vi "Calculate_Cost_F()-3.vi"(0 "[IN] Subtracks":T2(array[cluster]), 1 "[IN] Still connected\ntracks in group":T1, 2 "[IN] Max angle":dbl, 3 "[IN] Areas particles\nPrimary Detected":dbl[][](array[numeric]), 7 "[IN] Index of Earliest \nProblem Point Inside":i32, 9 "[IN] # of Longest track\nInside the Tracks Group":i32, 11 "error IN":errorcluster, 12 "[IN] Primary \n(X,Y) Detected":dbl[][](array[numeric]), 13 "[IN] Potentially\nMoving (X,Y)":dbl[][](array[numeric]), 14 "[IN] Dot matrix with statuses \nfor potentially moving dots":i16[][](array[numeric])) -> (4 "[OUT] Cost function":i8[](array[numeric]), 15 "error OUT":errorcluster)   [LabVIEW 2013]
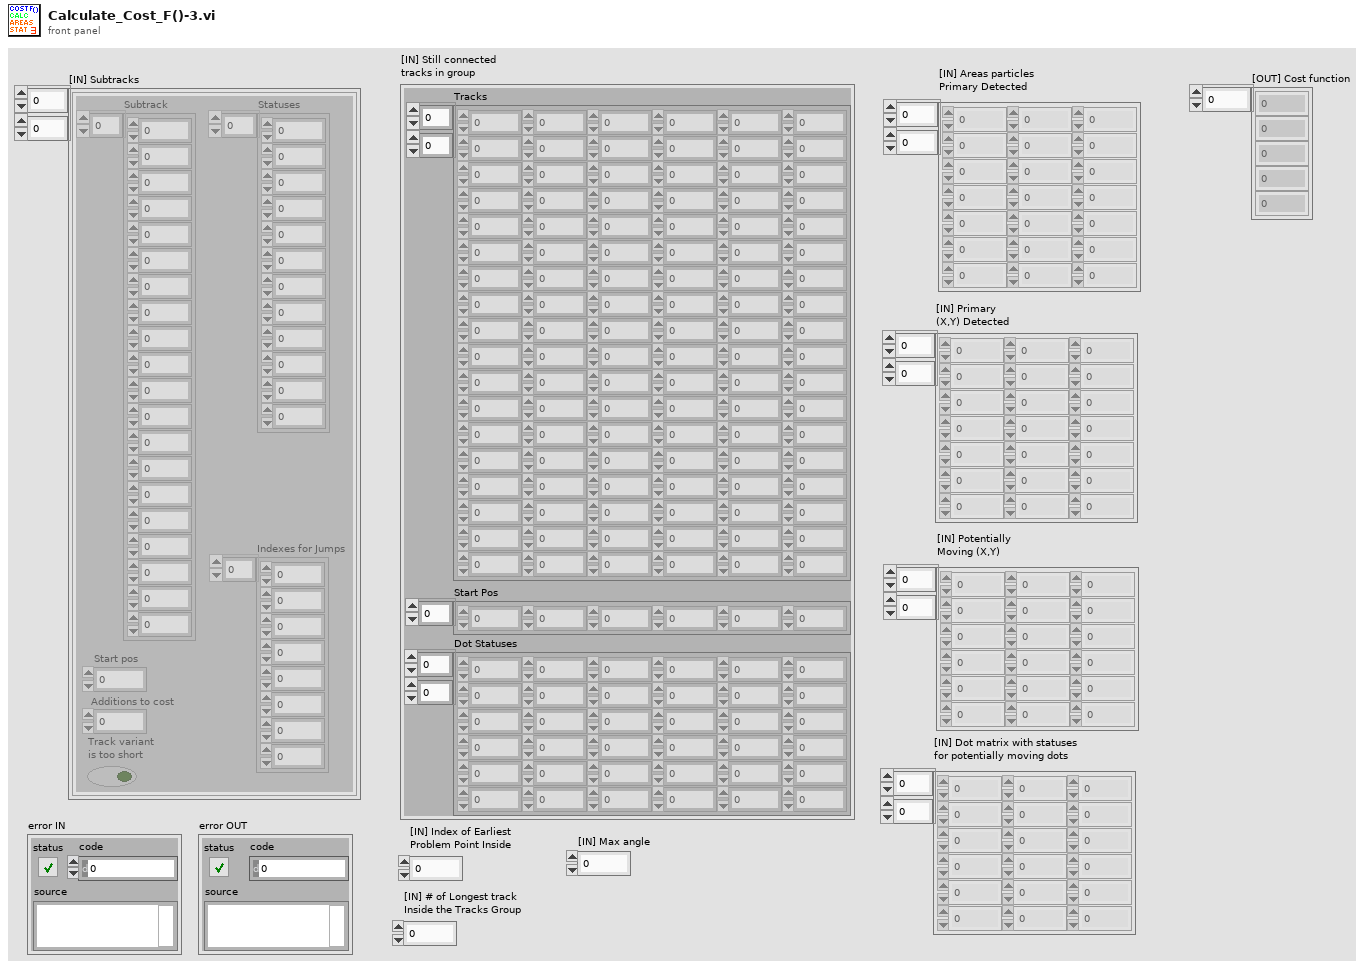
[diagram p1: front panel]
types:
  T1 = cluster{"Tracks":dbl[][], "Start Pos":i32[], "Dot Statuses":i16[][]}
  T2 = cluster{"Subtrack":dbl[], "Statuses":i16[], "Start pos":i32, "Additions to cost":i32, "Track variant \nis too short":bool, "Indexes for Jumps":i32[]}[][]
  T3 = cluster{"Subtrack":dbl[], "Statuses":i16[], "Start pos":i32, "Additions to cost":i32, "Track variant \nis too short":bool, "Indexes for Jumps":i32[]}[]
  T4 = cluster{"Subtrack":dbl[], "Statuses":i16[], "Start pos":i32, "Additions to cost":i32, "Track variant \nis too short":bool, "Indexes for Jumps":i32[]}
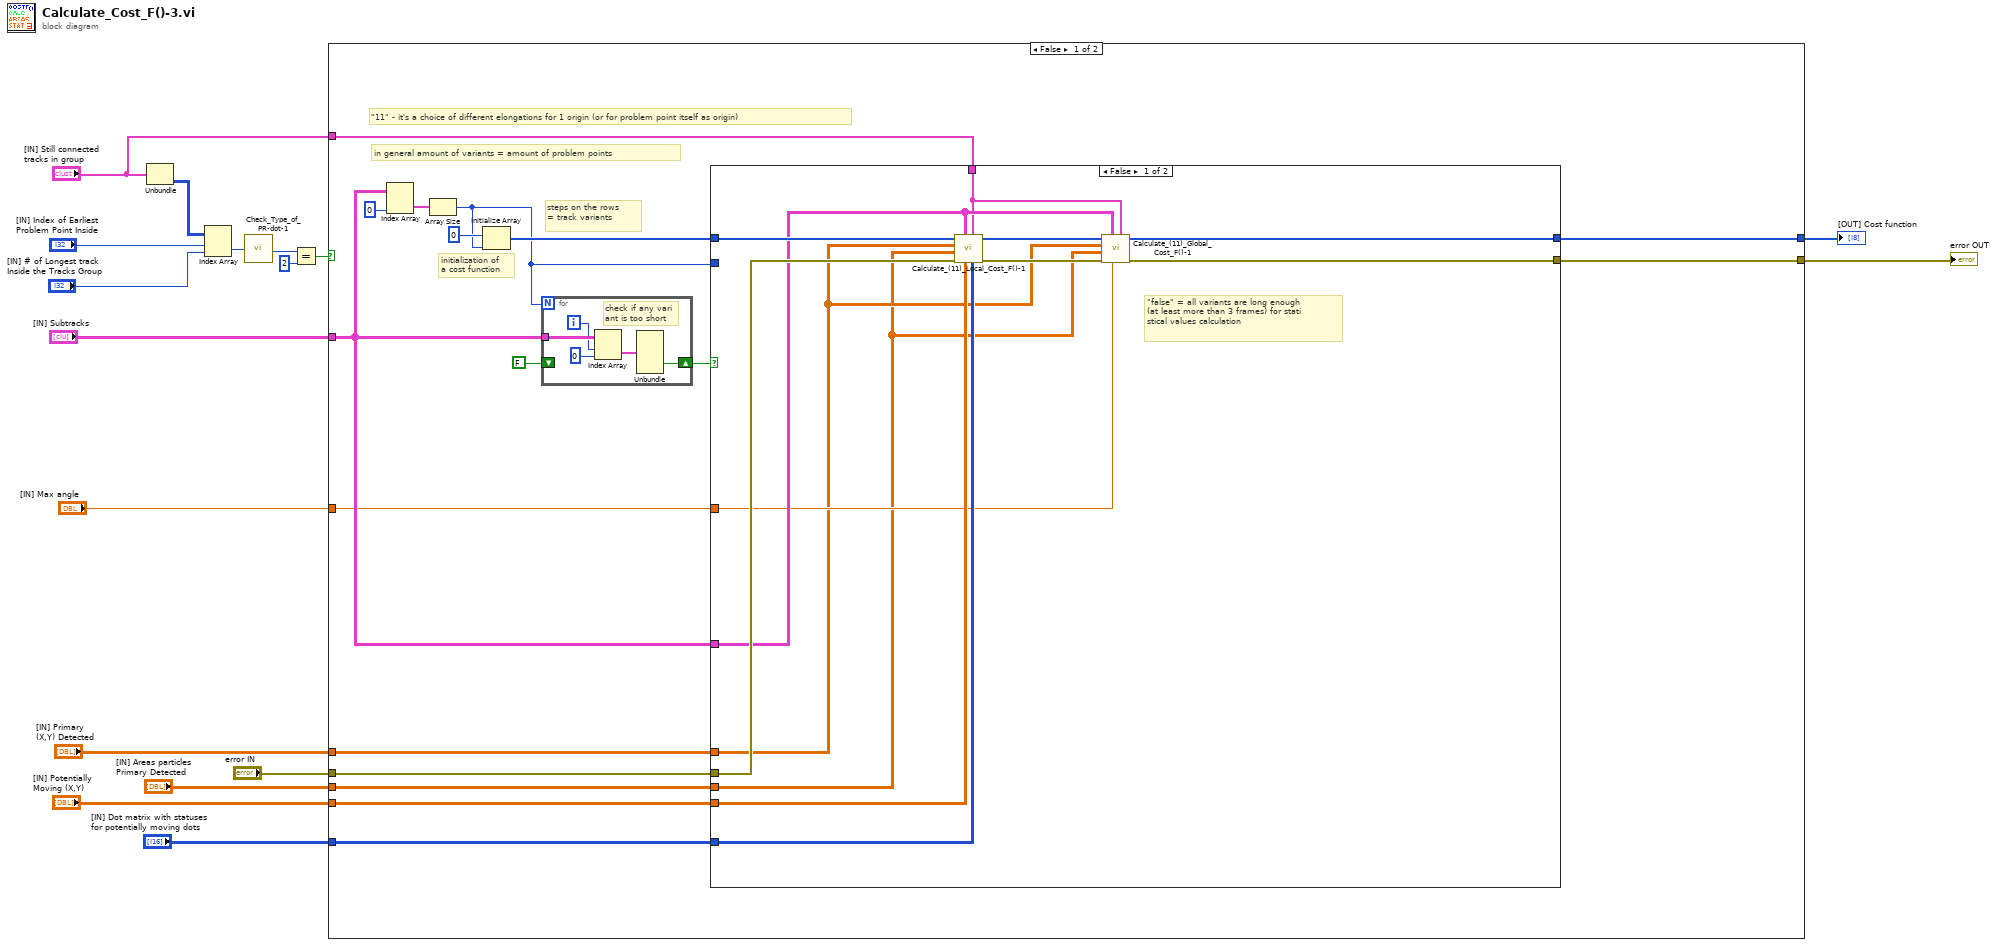
[diagram p0: block diagram]
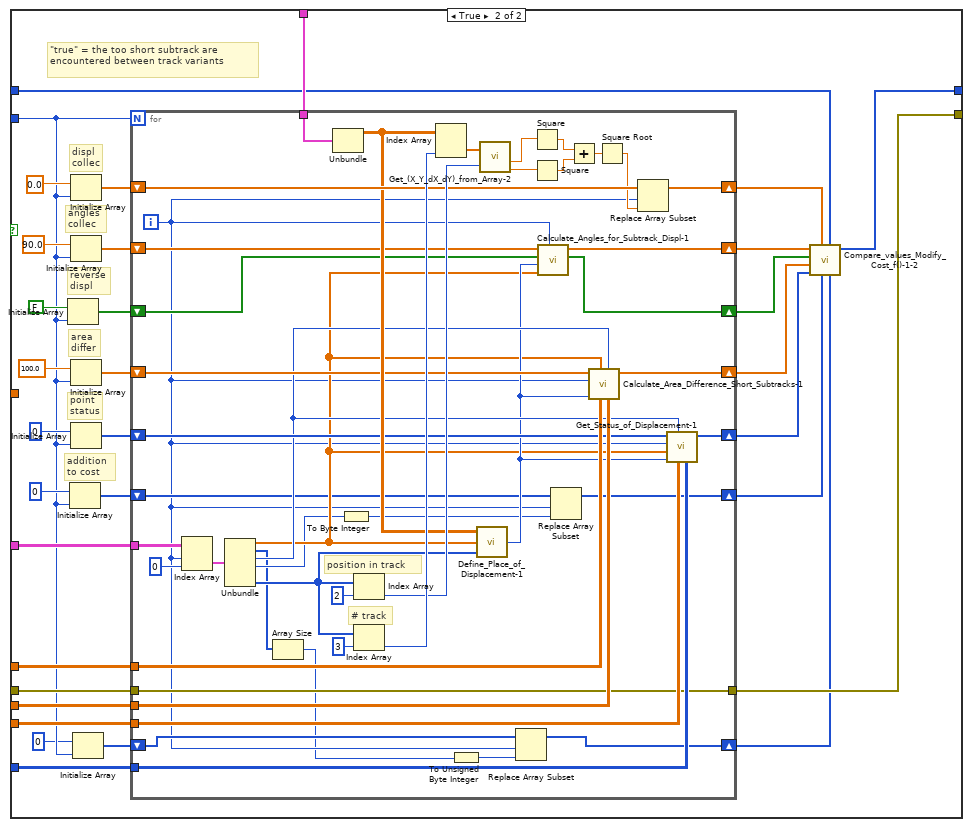
[diagram p2: hidden frame]
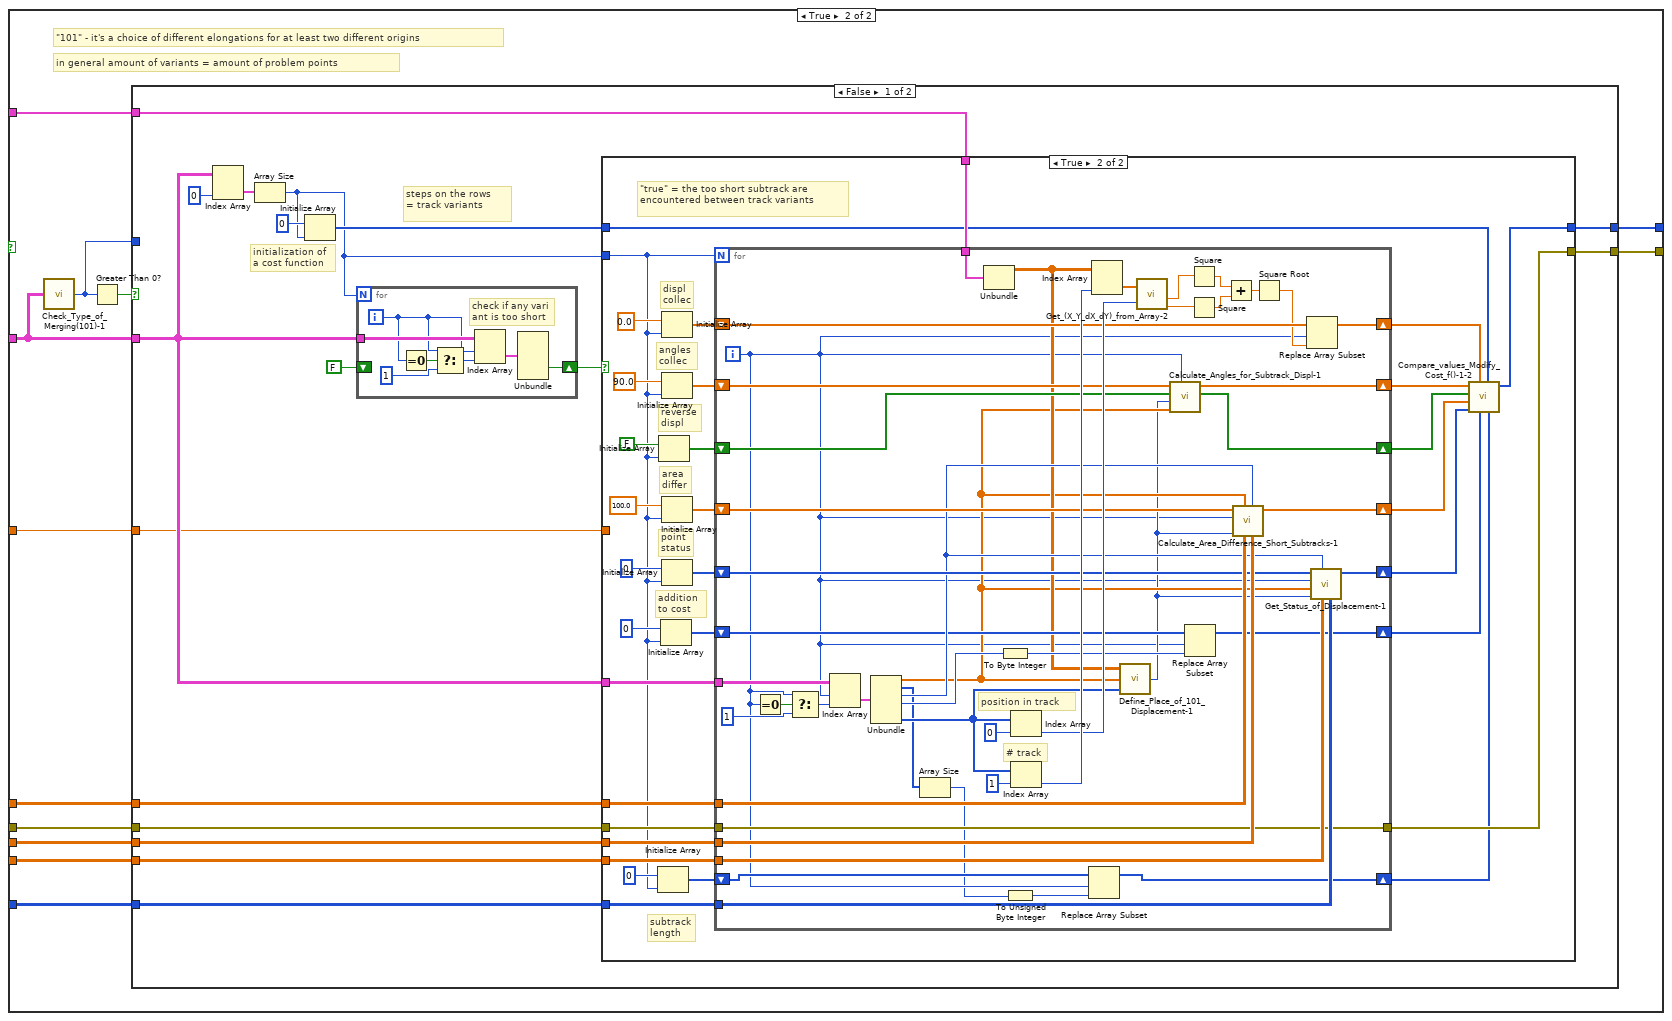
[diagram p3: hidden frame]
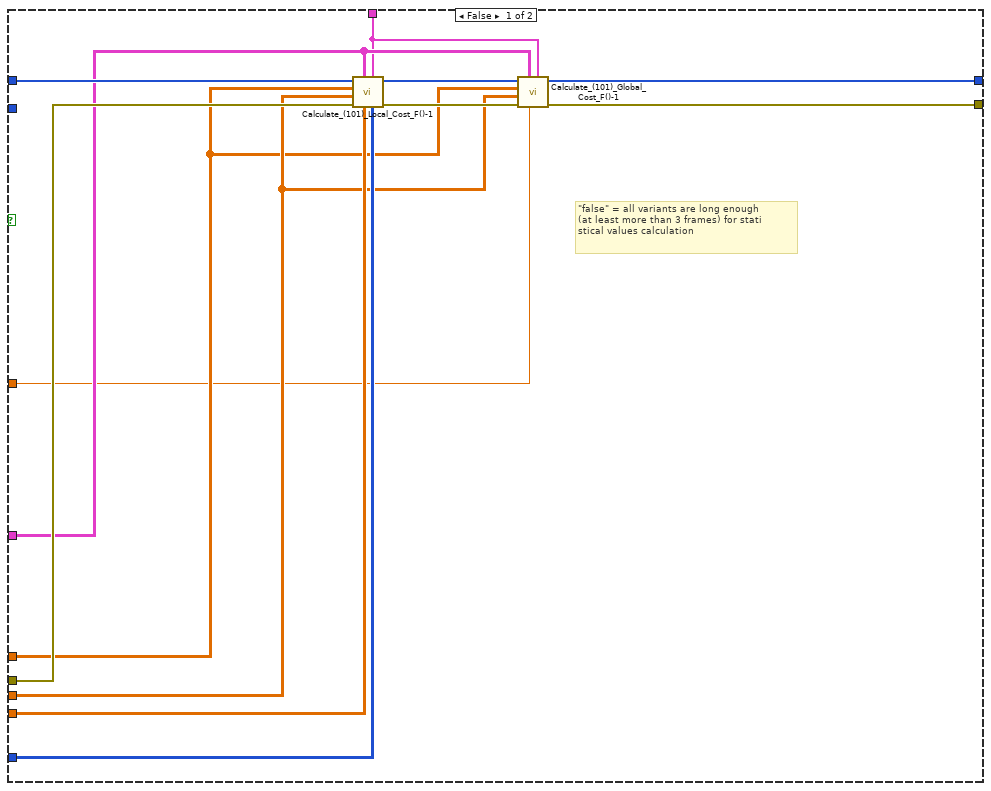
[diagram p4: hidden frame]
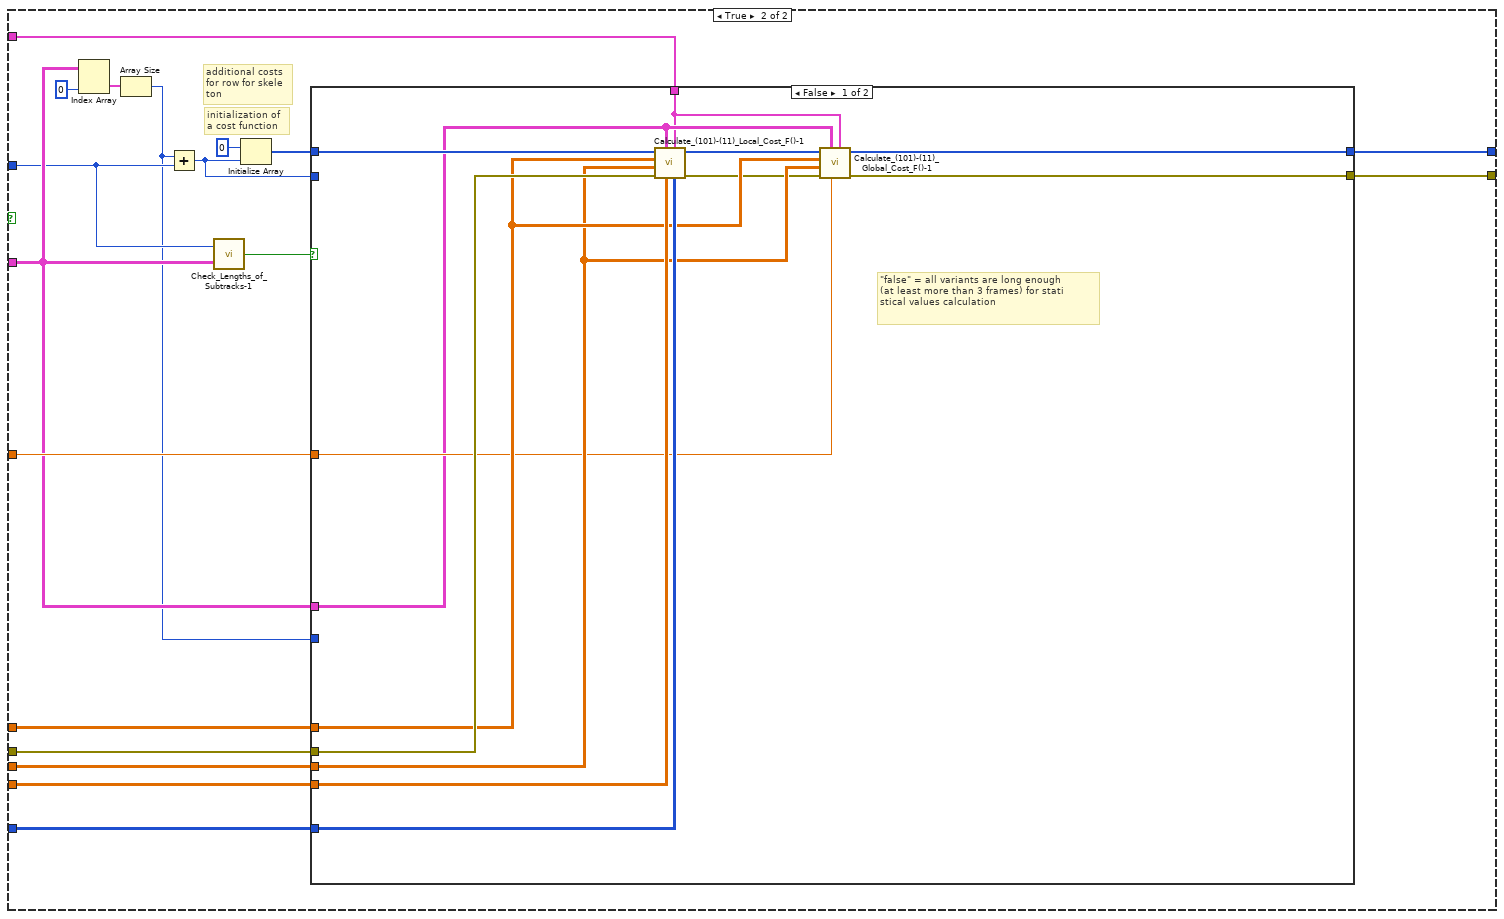
[diagram p5: hidden frame]
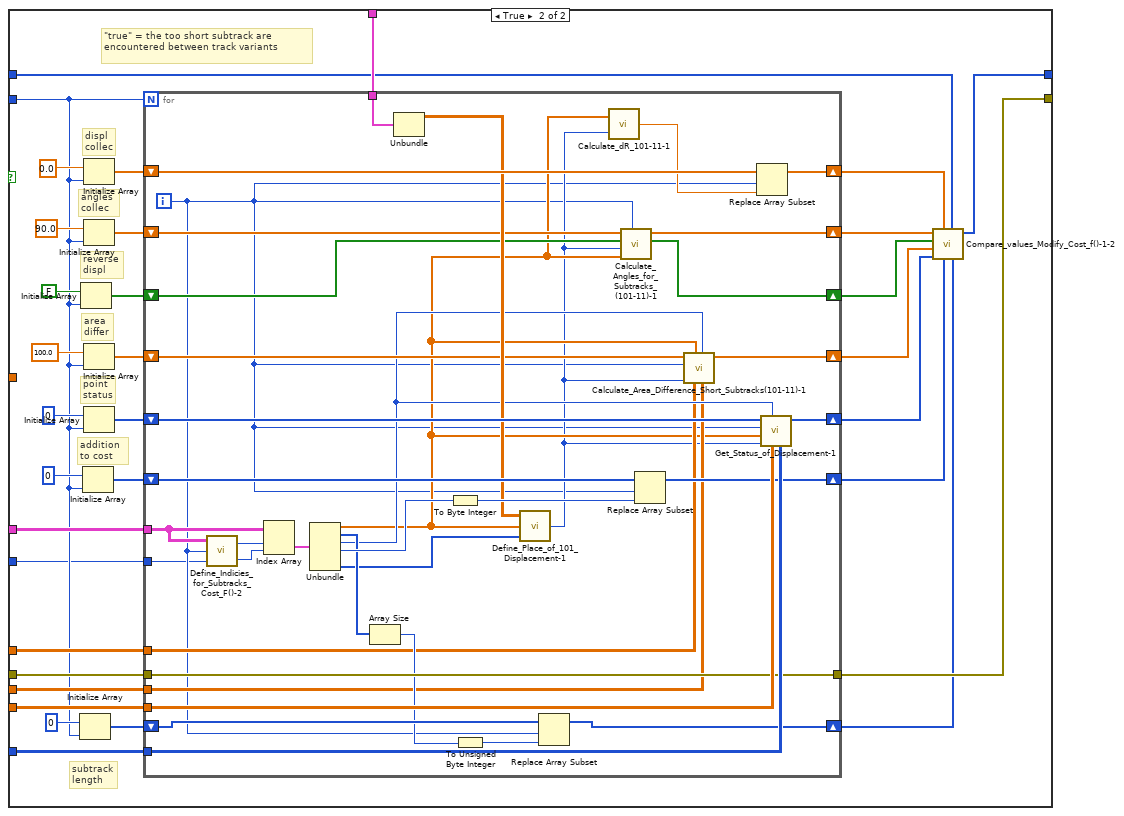
[diagram p6: hidden frame]
diagram:
  n1 = Unbundle("[IN] Still connected\ntracks in group") -> ("Dot Statuses"=w15:i16[][])  [unwired: 2 out]
  n2 = Index Array(array=w15, index (row)="[IN] Index of Earliest \nProblem Point Inside", index (col)="[IN] # of Longest track\nInside the Tracks Group") -> (element=w14:i16)
  n3 = call "Check_Type_of_PR-dot-1.vi"("[IN] dot status"=w14) -> ("[OUT] Type of\nproblem dot"=w17:i32)
  n4 = Equal?(x=w17, y=2) -> (x = y?=w13:bool)
  n5 = case shown="False" w13 {
    tunnel: "[IN] Subtracks" -> [w27 w133]
    tunnel: "[IN] Still connected\ntracks in group" -> [w26 w130]
    tunnel: "[IN] Primary \n(X,Y) Detected" -> [w25 w140]
    tunnel: "[IN] Areas particles\nPrimary Detected" -> [w24 w138]
    tunnel: "[IN] Potentially\nMoving (X,Y)" -> [w23 w137]
    tunnel: "[IN] Dot matrix with statuses \nfor potentially moving dots" -> [w22 w136]
    tunnel: "error IN" -> [w21 w139]
    tunnel: "[IN] Max angle" -> [w20 w141]
    tunnel: [w19 w135] -> w2
    tunnel: [w18 w134] -> w1
    frame False {
      # "initialization of \na cost function"
      # "steps on the rows\n= track variants"
      # "in general amount of variants = amount of problem points"
      # "\"11\" - it's a choice of different elongations for 1 origin (or for problem point itself as origin)"
      n6 = Index Array(array=w27, index (col)=0 ("disabled index (col)")) -> (element=w33:T3)  [unwired: 1 in]
      n7 = Array Size(array=w33) -> (size(s)=w28:i32)
      n8 = Initialize Array(i8 0, w28) -> (w29:i8[])
      n9 = for {
        N: w28 -> [_]
        tunnel: w27 -> [w129]
        shift-right: [w125] -> w30
        shift-left: FALSE -> [_]
        i -> [w126]
        # "check if any vari\nant is too short"
        n10 = Index Array(array=w129, index (row)=w126, index (col)=0 ("disabled index (col)")) -> (element=w127:T4)
        n11 = Unbundle(w127) -> ("Track variant \nis too short"=w125:bool)  [unwired: 5 out]
      }
      n12 = case shown="False" w30 {
        tunnel: w29 -> [w47 w54]
        tunnel: w28 -> [_ w59]
        tunnel: w27 -> [w42 w79]
        tunnel: w26 -> [w41 w78]
        tunnel: w25 -> [w38 w69]
        tunnel: w24 -> [w37 w68]
        tunnel: w23 -> [w45 w65]
        tunnel: w22 -> [w44 w64]
        tunnel: w21 -> [w46 w61]
        tunnel: w20 -> [w39 _]
        tunnel: [w36 w53] -> w19
        tunnel: [w35 w60] -> w18
        frame False {
          # "\"false\" = all variants are long enough\n(at least more than 3 frames) for stati\nstical values calculation"
          n13 = call "Calculate_(11)_Local_Cost_F()-1.vi"("[IN] Dot matrix with statuses \nfor potentially moving dots"=w44, "[IN] Still connected\ntracks in group"=w41, "[IN] Potentially\nMoving (X,Y)"=w45, "[IN] Subtracks"=w42, "error IN"=w46, "[IN] Areas particles\nPrimary Detected"=w37, "[IN] Primary \n(X,Y) Detected"=w38, "[IN] Cost function"=w47) -> ("error OUT"=w40:errorcluster, "[OUT] Cost function"=w43:i8[])  [unwired: 2 in]
          n14 = call "Calculate_(11)_Global_Cost_F()-1.vi"("[IN] Still connect\ned tracks in group"=w41, "[IN] Max angle"=w39, "[IN] Subtracks"=w42, "error IN"=w40, "[IN] Areas particles\nPrimary Detected"=w37, "[IN] Primary \n(X,Y) Detected"=w38, "[IN] Cost function"=w43) -> ("error OUT"=w35:errorcluster, "[OUT] Cost function"=w36:i8[])  [unwired: 3 in]
        }
        frame True {
          # "addition \nto cost"
          # "point\nstatus"
          # "area \ndiffer"
          # "reverse \ndispl"
          # "angles \ncollec"
          # "displ \ncollec"
          # "\"true\" = the too short subtrack are \nencountered between track variants"
          n15 = Initialize Array(FALSE, w59) -> (w72:bool[])
          n16 = Initialize Array(i8 0, w59) -> (w62:i8[])
          n17 = Initialize Array(0.0, w59) -> (w76:dbl[])
          n18 = Initialize Array(90.0, w59) -> (w74:dbl[])
          n19 = Initialize Array(100.0, w59) -> (w70:dbl[])
          n20 = Initialize Array(i16 0, w59) -> (w66:i16[])
          n21 = Initialize Array(u8 0, w59) -> (w57:u8[])
          n22 = for {
            N: w59 -> [_]
            tunnel: w79 -> [w124]
            tunnel: w78 -> [w119]
            shift-right: [w114] -> w55
            shift-left: w76 -> [w115]
            shift-right: [w110] -> w56
            shift-left: w74 -> [w111]
            shift-right: [w108] -> w52
            shift-left: w72 -> [w109]
            tunnel: w69 -> [w104]
            tunnel: w68 -> [w106]
            shift-right: [w105] -> w51
            shift-left: w70 -> [w107]
            tunnel: w65 -> [w99]
            tunnel: w64 -> [w98]
            shift-right: [w97] -> w50
            shift-left: w66 -> [w103]
            shift-right: [w93] -> w49
            shift-left: w62 -> [w96]
            tunnel: w61 -> [w86]
            tunnel: [w86] -> w60
            shift-right: [w83] -> w48
            shift-left: w57 -> [w84]
            i -> [w82]
            # "# track"
            # "position in track"
            n23 = Index Array(array=w124, index (row)=w82, index (col)=0 ("disabled index (col)")) -> (element=w122:T4)
            n24 = Unbundle(w122) -> ("Subtrack"=w100:dbl[], "Statuses"=w85:i16[], "Start pos"=w102:i32, "Additions to cost"=w95:i32, "Indexes for Jumps"=w112:i32[])  [unwired: 1 out]
            n25 = Array Size(array=w85) -> (size(s)=w81:i32)
            n26 = Unbundle(w119) -> ("Tracks"=w113:dbl[][])  [unwired: 2 out]
            n27 = To Byte Integer(number=w95) -> (8bit integer=w94:i8)
            n28 = Index Array(array=w112, index=2) -> (element=w116:i32)
            n29 = Index Array(array=w112, index=3) -> (element=w118:i32)
            n30 = Index Array(array=w113, index (col)=w118) -> (element=w117:dbl[])  [unwired: 1 in]
            n31 = To Unsigned Byte Integer(number=w81) -> (unsigned 8bit integer=w80:u8)
            n32 = call "Define_Place_of_Displacement-1.vi"("[IN] Indexes for Jumps"=w112, "[IN] Subtrack"=w100, "[IN] Tracks"=w113) -> ("[OUT] Index of \"11\" Dis\nplacement in Subtrack"=w101:i32)  [unwired: 2 in]
            n33 = call "Get_(X_Y_dX_dY)_from_Array-2.vi"("(X,Y,dX,dY)"=w117, "Index of Displacement"=w116) -> ("dX"=w89:dbl, "dY"=w88:dbl)  [unwired: 2 out]
            n34 = Replace Array Subset(array=w84, new element=w80, index=w82) -> (w83:u8[])
            n35 = Square(x=w89) -> (x^2=w92:dbl)
            n36 = Square(x=w88) -> (x^2=w91:dbl)
            n37 = call "Calculate_Angles_for_Subtrack_Displ-1.vi"("[IN] Index of subtrack"=w82, "[IN] Subtrack"=w100, "[IN] Index of \"11\" Dis-\nplacement in Subtrack"=w101, "[IN] Reverse Displ or Not"=w109, "[IN] Array with Angles \nBetween Displacement"=w111) -> ("[OUT] Reverse displacement or not"=w108:bool[], "[OUT] Angles betwe\nen two displacements"=w110:dbl[])  [unwired: 3 in]
            n38 = Replace Array Subset(array=w96, new element=w94, index=w82) -> (w93:i8[])
            n39 = Add(x=w92, y=w91) -> (x+y=w90:dbl)
            n40 = call "Calculate_Area_Difference_Short_Subtracks-1.vi"("[IN] Areas particles\nPrimary Detected"=w106, "[IN] Start pos"=w102, "[IN] Primary \n(X,Y) Detected"=w104, "[IN] Subtrack"=w100, "[IN] Index of \"11\" Dis-\nplacement in Subtrack"=w101, "[IN] Index of\n subtrack"=w82, "[IN] Areas \ndifference"=w107) -> ("[OUT] Areas \ndifference"=w105:dbl[])  [unwired: 4 in]
            n41 = Square Root(x=w90) -> (sqrt(x)=w87:dbl)
            n42 = Replace Array Subset(array=w115, new element=w87, index=w82) -> (w114:dbl[])
            n43 = call "Get_Status_of_Displacement-1.vi"("[IN] Dot matrix with statuses\nfor potentially moving dots"=w98, "[IN] Potentially\nMoving (X,Y)"=w99, "[IN] Start pos"=w102, "[IN] Index of Problem\nPoint in Subtrack"=w101, "[IN] Subtrack"=w100, "[IN] Index of\n subtrack"=w82, "[IN] Displace-\nment Statuses"=w103) -> ("[OUT] Displace\nment Statuses"=w97:i16[])  [unwired: 4 in]
          }
          n44 = call "Compare_values_Modify_Cost_f()-1-2.vi"("[IN] Track Length"=w48, "[IN] Cost function"=w54, "[IN] Additions to cost"=w49, "[IN] Array of displa\ncement differences"=w55, "[IN] Statuses of points"=w50, "[IN] Areas \ndifferences"=w51, "[IN] Reverse or not"=w52, "[IN] Angles betwe\nen displacements"=w56) -> ("[OUT] Cost function"=w53:i8[])  [unwired: 3 in]
        }
      }
    }
    frame True {
      # "in general amount of variants = amount of problem points"
      # "\"101\" - it's a choice of different elongations for at least two different origins"
      n45 = call "Check_Type_of_Merging(101)-1.vi"("[IN] Subtracks"=w133) -> ("[OUT] # of Additional Costs"=w131:i32)
      n46 = Greater Than 0?(x=w131) -> (x > 0?=w132:bool)
      n47 = case shown="False" w132 {
        tunnel: w130 -> [w151 w265]
        tunnel: w133 -> [w150 w264]
        tunnel: w141 -> [w149 w266]
        tunnel: w140 -> [w148 w271]
        tunnel: w139 -> [w147 w270]
        tunnel: w138 -> [w146 w269]
        tunnel: w137 -> [w145 w268]
        tunnel: w136 -> [w144 w267]
        tunnel: [w143 w259] -> w135
        tunnel: [w142 w258] -> w134
        tunnel: w131 -> [_ w261]
        frame False {
          # "initialization of \na cost function"
          # "steps on the rows\n= track variants"
          n48 = Index Array(array=w150, index (col)=0 ("disabled index (col)")) -> (element=w157:T3)  [unwired: 1 in]
          n49 = Array Size(array=w157) -> (size(s)=w152:i32)
          n50 = Initialize Array(i8 0, w152) -> (w153:i8[])
          n51 = for {
            N: w152 -> [_]
            tunnel: w150 -> [w257]
            shift-right: [w255] -> w154
            shift-left: FALSE -> [_]
            i -> [w251]
            # "check if any vari\nant is too short"
            n52 = Equal To 0?(x=w251) -> (x = 0?=w254:bool)
            n53 = Select(t=w251, s=w254, f=1) -> (s? t:f=w252:i32)
            n54 = Index Array(array=w257, index (row)=w251, index (col)=w252) -> (element=w256:T4)
            n55 = Unbundle(w256) -> ("Track variant \nis too short"=w255:bool)  [unwired: 5 out]
          }
          n56 = case shown="True" w154 {
            tunnel: w153 -> [w171 w178]
            tunnel: w152 -> [_ w182]
            tunnel: w150 -> [w163 w203]
            tunnel: w151 -> [w162 w202]
            tunnel: w148 -> [w165 w193]
            tunnel: w146 -> [w166 w192]
            tunnel: w145 -> [w170 w189]
            tunnel: w144 -> [w168 w188]
            tunnel: w147 -> [w169 w185]
            tunnel: w149 -> [w161 _]
            tunnel: [w160 w177] -> w143
            tunnel: [w159 w184] -> w142
            frame False {
              # "\"false\" = all variants are long enough\n(at least more than 3 frames) for stati\nstical values calculation"
              n57 = call "Calculate_(101)_Local_Cost_F()-1.vi"("[IN] Dot matrix with statuses \nfor potentially moving dots"=w168, "[IN] Still connected\ntracks in group"=w162, "[IN] Potentially\nMoving (X,Y)"=w170, "[IN] Subtracks"=w163, "error IN"=w169, "[IN] Areas particles\nPrimary Detected"=w166, "[IN] Primary \n(X,Y) Detected"=w165, "[IN] Cost function"=w171) -> ("error OUT"=w167:errorcluster, "[OUT] Cost function"=w164:i8[])  [unwired: 2 in]
              n58 = call "Calculate_(101)_Global_Cost_F()-1.vi"("[IN] Still connect\ned tracks in group"=w162, "[IN] Max angle"=w161, "[IN] Subtracks"=w163, "error IN"=w167, "[IN] Areas particles\nPrimary Detected"=w166, "[IN] Primary \n(X,Y) Detected"=w165, "[IN] Cost function"=w164) -> ("error OUT"=w159:errorcluster, "[OUT] Cost function"=w160:i8[])  [unwired: 3 in]
            }
            frame True {
              # "subtrack\nlength"
              # "addition \nto cost"
              # "point\nstatus"
              # "area \ndiffer"
              # "reverse \ndispl"
              # "angles \ncollec"
              # "displ \ncollec"
              # "\"true\" = the too short subtrack are \nencountered between track variants"
              n59 = Initialize Array(u8 0, w182) -> (w181:u8[])
              n60 = Initialize Array(FALSE, w182) -> (w196:bool[])
              n61 = Initialize Array(i8 0, w182) -> (w186:i8[])
              n62 = Initialize Array(0.0, w182) -> (w200:dbl[])
              n63 = Initialize Array(90.0, w182) -> (w198:dbl[])
              n64 = Initialize Array(100.0, w182) -> (w194:dbl[])
              n65 = Initialize Array(i16 0, w182) -> (w190:i16[])
              n66 = for {
                N: w182 -> [_]
                tunnel: w203 -> [w250]
                tunnel: w202 -> [w246]
                shift-right: [w241] -> w179
                shift-left: w200 -> [w242]
                shift-right: [w239] -> w180
                shift-left: w198 -> [w240]
                shift-right: [w237] -> w173
                shift-left: w196 -> [w238]
                tunnel: w193 -> [w233]
                tunnel: w192 -> [w235]
                shift-right: [w234] -> w174
                shift-left: w194 -> [w236]
                tunnel: w189 -> [w230]
                tunnel: w188 -> [w229]
                shift-right: [w228] -> w175
                shift-left: w190 -> [w232]
                shift-right: [w224] -> w176
                shift-left: w186 -> [w227]
                tunnel: w185 -> [w217]
                tunnel: [w217] -> w184
                shift-right: [w206] -> w172
                shift-left: w181 -> [w208]
                i -> [w207]
                # "# track"
                # "position in track"
                n67 = Equal To 0?(x=w207) -> (x = 0?=w216:bool)
                n68 = Select(t=w207, s=w216, f=1) -> (s? t:f=w214:i32)
                n69 = Index Array(array=w250, index (row)=w207, index (col)=w214) -> (element=w249:T4)
                n70 = Unbundle(w249) -> ("Subtrack"=w212:dbl[], "Statuses"=w209:i16[], "Start pos"=w231:i32, "Additions to cost"=w226:i32, "Indexes for Jumps"=w211:i32[])  [unwired: 1 out]
                n71 = Array Size(array=w209) -> (size(s)=w205:i32)
                n72 = Unbundle(w246) -> ("Tracks"=w213:dbl[][])  [unwired: 2 out]
                n73 = To Byte Integer(number=w226) -> (8bit integer=w225:i8)
                n74 = To Unsigned Byte Integer(number=w205) -> (unsigned 8bit integer=w204:u8)
                n75 = Index Array(array=w211, index=0) -> (element=w243:i32)
                n76 = Index Array(array=w211, index=1) -> (element=w245:i32)
                n77 = Replace Array Subset(array=w208, new element=w204, index=w207) -> (w206:u8[])
                n78 = Index Array(array=w213, index (col)=w245) -> (element=w244:dbl[])  [unwired: 1 in]
                n79 = call "Define_Place_of_101_Displacement-1.vi"("[IN] Indexes for Jumps"=w211, "[IN] Subtrack"=w212, "[IN] Tracks"=w213) -> ("[OUT] Index of \"11\" Dis\nplacement in Subtrack"=w210:i32)  [unwired: 2 in]
                n80 = call "Get_(X_Y_dX_dY)_from_Array-2.vi"("(X,Y,dX,dY)"=w244, "Index of Displacement"=w243) -> ("dX"=w220:dbl, "dY"=w219:dbl)  [unwired: 2 out]
                n81 = call "Calculate_Angles_for_Subtrack_Displ-1.vi"("[IN] Index of subtrack"=w207, "[IN] Subtrack"=w212, "[IN] Index of \"11\" Dis-\nplacement in Subtrack"=w210, "[IN] Reverse Displ or Not"=w238, "[IN] Array with Angles \nBetween Displacement"=w240) -> ("[OUT] Reverse displacement or not"=w237:bool[], "[OUT] Angles betwe\nen two displacements"=w239:dbl[])  [unwired: 3 in]
                n82 = Replace Array Subset(array=w227, new element=w225, index=w207) -> (w224:i8[])
                n83 = Square(x=w220) -> (x^2=w223:dbl)
                n84 = Square(x=w219) -> (x^2=w222:dbl)
                n85 = Add(x=w223, y=w222) -> (x+y=w221:dbl)
                n86 = call "Calculate_Area_Difference_Short_Subtracks-1.vi"("[IN] Areas particles\nPrimary Detected"=w235, "[IN] Start pos"=w231, "[IN] Primary \n(X,Y) Detected"=w233, "[IN] Subtrack"=w212, "[IN] Index of \"11\" Dis-\nplacement in Subtrack"=w210, "[IN] Index of\n subtrack"=w207, "[IN] Areas \ndifference"=w236) -> ("[OUT] Areas \ndifference"=w234:dbl[])  [unwired: 4 in]
                n87 = Square Root(x=w221) -> (sqrt(x)=w218:dbl)
                n88 = Replace Array Subset(array=w242, new element=w218, index=w207) -> (w241:dbl[])
                n89 = call "Get_Status_of_Displacement-1.vi"("[IN] Dot matrix with statuses\nfor potentially moving dots"=w229, "[IN] Potentially\nMoving (X,Y)"=w230, "[IN] Start pos"=w231, "[IN] Index of Problem\nPoint in Subtrack"=w210, "[IN] Subtrack"=w212, "[IN] Index of\n subtrack"=w207, "[IN] Displace-\nment Statuses"=w232) -> ("[OUT] Displace\nment Statuses"=w228:i16[])  [unwired: 4 in]
              }
              n90 = call "Compare_values_Modify_Cost_f()-1-2.vi"("[IN] Track Length"=w172, "[IN] Cost function"=w178, "[IN] Additions to cost"=w176, "[IN] Array of displa\ncement differences"=w179, "[IN] Statuses of points"=w175, "[IN] Areas \ndifferences"=w174, "[IN] Reverse or not"=w173, "[IN] Angles betwe\nen displacements"=w180) -> ("[OUT] Cost function"=w177:i8[])  [unwired: 3 in]
            }
          }
        }
        frame True {
          # "additional costs\nfor row for skele\nton"
          # "initialization of \na cost function"
          n91 = Index Array(array=w264, index (col)=0 ("disabled index (col)")) -> (element=w274:T3)  [unwired: 1 in]
          n92 = Array Size(array=w274) -> (size(s)=w260:i32)
          n93 = Add(x=w260, y=w261) -> (x+y=w262:i32)
          n94 = call "Check_Lengths_of_Subtracks-1.vi"("[IN] Subtracks"=w264, "[IN] Number of Additi\nonal Costs (Subtracks)"=w261) -> ("[OUT[ Is between subtracks\npresented too short one?"=w263:bool)
          n95 = Initialize Array(i8 0, w262) -> (w272:i8[])
          n96 = case shown="False" w263 {
            tunnel: w272 -> [w287 w296]
            tunnel: w262 -> [_ w300]
            tunnel: w264 -> [w279 w321]
            tunnel: w265 -> [w278 w320]
            tunnel: w271 -> [w283 w311]
            tunnel: w269 -> [w282 w310]
            tunnel: w268 -> [w286 w307]
            tunnel: w267 -> [w285 w306]
            tunnel: w270 -> [w288 w303]
            tunnel: w266 -> [w280 _]
            tunnel: [w277 w295] -> w259
            tunnel: [w276 w302] -> w258
            tunnel: w260 -> [_ w289]
            frame False {
              # "\"false\" = all variants are long enough\n(at least more than 3 frames) for stati\nstical values calculation"
              n97 = call "Calculate_(101)-(11)_Local_Cost_F()-1.vi"("[IN] Dot matrix with statuses \nfor potentially moving dots"=w285, "[IN] Still connected\ntracks in group"=w278, "[IN] Potentially\nMoving (X,Y)"=w286, "[IN] Subtracks"=w279, "error IN"=w288, "[IN] Areas particles\nPrimary Detected"=w282, "[IN] Primary \n(X,Y) Detected"=w283, "[IN] Cost function"=w287) -> ("error OUT"=w281:errorcluster, "[OUT] Cost function"=w284:i8[])  [unwired: 2 in]
              n98 = call "Calculate_(101)-(11)_Global_Cost_F()-1.vi"("[IN] Still connect\ned tracks in group"=w278, "[IN] Max angle"=w280, "[IN] Subtracks"=w279, "error IN"=w281, "[IN] Areas particles\nPrimary Detected"=w282, "[IN] Primary \n(X,Y) Detected"=w283, "[IN] Cost function"=w284) -> ("error OUT"=w276:errorcluster, "[OUT] Cost function"=w277:i8[])  [unwired: 3 in]
            }
            frame True {
              # "subtrack\nlength"
              # "addition \nto cost"
              # "point\nstatus"
              # "area \ndiffer"
              # "reverse \ndispl"
              # "angles \ncollec"
              # "displ \ncollec"
              # "\"true\" = the too short subtrack are \nencountered between track variants"
              n99 = Initialize Array(u8 0, w300) -> (w299:u8[])
              n100 = Initialize Array(FALSE, w300) -> (w314:bool[])
              n101 = Initialize Array(i8 0, w300) -> (w304:i8[])
              n102 = Initialize Array(0.0, w300) -> (w318:dbl[])
              n103 = Initialize Array(90.0, w300) -> (w316:dbl[])
              n104 = Initialize Array(100.0, w300) -> (w312:dbl[])
              n105 = Initialize Array(i16 0, w300) -> (w308:i16[])
              n106 = for {
                N: w300 -> [_]
                tunnel: w321 -> [w326]
                tunnel: w320 -> [w357]
                shift-right: [w355] -> w297
                shift-left: w318 -> [w356]
                shift-right: [w334] -> w298
                shift-left: w316 -> [w337]
                shift-right: [w335] -> w291
                shift-left: w314 -> [w336]
                tunnel: w311 -> [w329]
                tunnel: w310 -> [w330]
                shift-right: [w331] -> w292
                shift-left: w312 -> [w333]
                tunnel: w307 -> [w353]
                tunnel: w306 -> [w352]
                shift-right: [w351] -> w293
                shift-left: w308 -> [w354]
                shift-right: [w347] -> w294
                shift-left: w304 -> [w350]
                tunnel: w303 -> [w346]
                tunnel: [w346] -> w302
                shift-right: [w344] -> w290
                shift-left: w299 -> [w345]
                tunnel: w289 -> [w322]
                i -> [w323]
                n107 = call "Define_Indicies_for_Subtracks_Cost_F()-2.vi"("[IN] Number of Rows"=w322, "[IN] Current index"=w323, "[IN] Subtracks"=w326) -> ("[OUT] Column \n# for Subtrack"=w324:i32, "[OUT] Row # \nfor Subtrack"=w325:i32)
                n108 = Index Array(array=w326, index (row)=w325, index (col)=w324) -> (element=w358:T4)
                n109 = Unbundle(w358) -> ("Subtrack"=w328:dbl[], "Statuses"=w340:i16[], "Start pos"=w332:i32, "Additions to cost"=w349:i32, "Indexes for Jumps"=w339:i32[])  [unwired: 1 out]
                n110 = Array Size(array=w340) -> (size(s)=w343:i32)
                n111 = Unbundle(w357) -> ("Tracks"=w341:dbl[][])  [unwired: 2 out]
                n112 = To Byte Integer(number=w349) -> (8bit integer=w348:i8)
                n113 = To Unsigned Byte Integer(number=w343) -> (unsigned 8bit integer=w342:u8)
                n114 = call "Define_Place_of_101_Displacement-1.vi"("[IN] Indexes for Jumps"=w339, "[IN] Subtrack"=w328, "[IN] Tracks"=w341) -> ("[OUT] Index of \"11\" Dis\nplacement in Subtrack"=w327:i32)  [unwired: 2 in]
                n115 = Replace Array Subset(array=w345, new element=w342, index=w323) -> (w344:u8[])
                n116 = call "Calculate_dR_101-11-1.vi"("[IN] Index of \"101\"\nDisplacement"=w327, "[IN] Subtrack"=w328) -> ("[OUT] Displacement average"=w338:dbl)
                n117 = call "Calculate_Angles_for_Subtracks_(101-11)-1.vi"("[IN] Index of subtrack"=w323, "[IN] Subtrack"=w328, "[IN] Index of \"101\" Dis-\nplacement in Subtrack"=w327, "[IN] Reverse Displ or Not"=w336, "[IN] Array with Angles \nBetween Displacement"=w337) -> ("[OUT] Reverse displacement or not"=w335:bool[], "[OUT] Angles betwe\nen two displacements"=w334:dbl[])  [unwired: 3 in]
                n118 = Replace Array Subset(array=w350, new element=w348, index=w323) -> (w347:i8[])
                n119 = call "Calculate_Area_Difference_Short_Subtracks(101-11)-1.vi"("[IN] Areas particles\nPrimary Detected"=w330, "[IN] Start pos"=w332, "[IN] Primary \n(X,Y) Detected"=w329, "[IN] Subtrack"=w328, "[IN] Index of \"101\" Dis-\nplacement in Subtrack"=w327, "[IN] Index of\n subtrack"=w323, "[IN] Areas \ndifference"=w333) -> ("[OUT] Areas differen\nce (101 + 11 points)"=w331:dbl[])  [unwired: 4 in]
                n120 = Replace Array Subset(array=w356, new element=w338, index=w323) -> (w355:dbl[])
                n121 = call "Get_Status_of_Displacement-1.vi"("[IN] Dot matrix with statuses\nfor potentially moving dots"=w352, "[IN] Potentially\nMoving (X,Y)"=w353, "[IN] Start pos"=w332, "[IN] Index of Problem\nPoint in Subtrack"=w327, "[IN] Subtrack"=w328, "[IN] Index of\n subtrack"=w323, "[IN] Displace-\nment Statuses"=w354) -> ("[OUT] Displace\nment Statuses"=w351:i16[])  [unwired: 4 in]
              }
              n122 = call "Compare_values_Modify_Cost_f()-1-2.vi"("[IN] Track Length"=w290, "[IN] Cost function"=w296, "[IN] Additions to cost"=w294, "[IN] Array of displa\ncement differences"=w297, "[IN] Statuses of points"=w293, "[IN] Areas \ndifferences"=w292, "[IN] Reverse or not"=w291, "[IN] Angles betwe\nen displacements"=w298) -> ("[OUT] Cost function"=w295:i8[])  [unwired: 3 in]
            }
          }
        }
      }
    }
  }
  "error OUT" <- w1
  "[OUT] Cost function" <- w2
